vi "5v_to_16bit.vi"(11 "voltage":dbl) -> (3 "Bits":dbl)   [LabVIEW 2016]
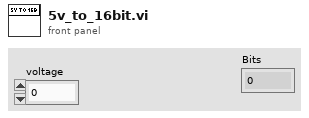
[diagram p1: front panel]
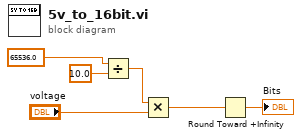
[diagram p0: block diagram]
diagram:
  n1 = Divide(x=65536.0, y=10.0) -> (x/y=w1:dbl)
  n2 = Multiply(x=w1, y="voltage") -> (x*y=w6:dbl)
  n3 = Round Toward +Infinity(x=w6) -> (ceil(x): smallest int >= x=→"Bits":dbl)
